vi "WaveformSimulator.vi"() -> ()   [LabVIEW 2015]
uses:
  <vilib>/imath/engines/lvmath2/RunTimeEngine/Managers/WorkSpace/UID Generator.vi
  <vilib>/imath/engines/lvmath2/RunTimeEngine/RunTimeType/NIMS_RunTimeType_From StrictType (excl LVString).vi
  <instcachedir>/0/NIMS_RunTimeType_From StrictType (excl LVString)_EB1C38A9BC5048DA9ABDA8F781E54D21.lvgen/NIMS_RunTimeType_From StrictType (excl LVString)_EB1C38A9BC5048DA9ABDA8F781E54D21_000.vi
  <vilib>/imath/engines/lvmath2/RunTimeEngine/LocalVariableDefStatement/MC_LocalVariableDefStatement_Display.vi
  <vilib>/imath/engines/lvmath2/RunTimeEngine/RangeToken/NIMS_Range.vi
  <instcachedir>/0/NIMS_Range_D919CC09935940E88F755EC1C6F49AC1.lvgen/NIMS_Range_D919CC09935940E88F755EC1C6F49AC1_000.vi
  <vilib>/imathl/engines/lvmath/Functions/Error Handling/Create Error.vi
  <vilib>/imath/engines/lvmath2/RunTimeEngine/ArithmeticOperatorToken/NIMS_ArithmeticOperator_plus.vi
  <instcachedir>/0/NIMS_ArithmeticOperator_plus_A4F2756F5ADB4A0090E0DBD7C10701C8.lvgen/NIMS_ArithmeticOperator_plus_A4F2756F5ADB4A0090E0DBD7C10701C8_004.vi
  <vilib>/imath/engines/lvmath2/RunTimeEngine/BuiltInFunctions/gensignal/NIMS_gensignal(str,RS,RS,RS).vi
  <vilib>/imath/engines/lvmath2/RunTimeEngine/BuiltInFunctions/linramp/NIMS_linramp.vi
  <vilib>/imath/engines/lvmath2/RunTimeEngine/VariableToken/NIMS_VariableToken_CondDefined.vi
  <instcachedir>/0/NIMS_VariableToken_CondDefined_FE30D0A1BFB24F098D41DEBABFE96BE1.lvgen/NIMS_VariableToken_CondDefined_FE30D0A1BFB24F098D41DEBABFE96BE1_001.vi
  <vilib>/imath/engines/lvmath2/RunTimeEngine/NodeEndStatement/NIMS_NodeEndStatement_Get Vector.vi
  <instcachedir>/0/NIMS_NodeEndStatement_Get Vector_ED7FC4F6B50246F79D573C75B2E51AF8.lvgen/NIMS_NodeEndStatement_Get Vector_ED7FC4F6B50246F79D573C75B2E51AF8_001.vi
  <vilib>/imath/engines/lvmath/Functions/Error Handling/MergeErrorsWrapper.vi
  <vilib>/imath/engines/lvmath2/RunTimeEngine/Managers/SymbolTable/Clear UID.vi
  <vilib>/imath/engines/lvmath2/RunTimeEngine/NodeEndStatement/NIMS_NodeEndStatement_Output.vi
  <instcachedir>/0/NIMS_NodeEndStatement_Output_53EC0D466D134D7ABD903AC30B43404B.lvgen/NIMS_NodeEndStatement_Output_53EC0D466D134D7ABD903AC30B43404B_005.vi
  <vilib>/imath/engines/lvmath2/RunTimeEngine/ErrorHandling/NIMS_Finalize Error.vi
  <vilib>/imath/engines/lvmath2/RunTimeEngine/Managers/SymbolTable/NIMS_WorkSpace.lvlib
panel:
  out "Waveform Output":cluster{"Time":dbl[], "Displacement":dbl[]} {"Displacement" format="%#_13g"; "Time" format="%#_13g"}
  in  "Waveform Parameters":T1
  in  "Digitizing Parameters":T2
  out "XY Graph":cluster{"t":dbl[], "x":dbl[]}(graph)
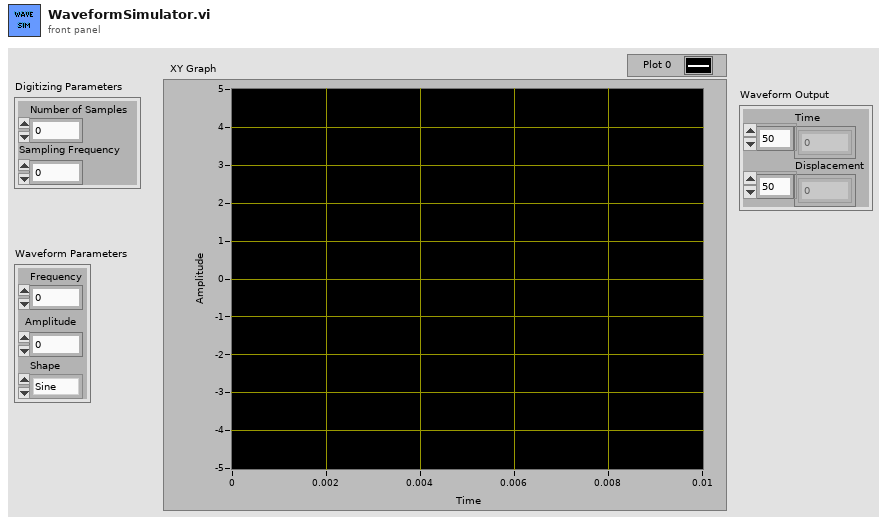
[diagram p1: front panel]
types:
  T1 = cluster{"Frequency":i32, "Amplitude":i32, "Shape":enum16{"Sine", "Cosine", "LinRamp", "Square", "SineCosine"}}
  T2 = cluster{"Number of Samples":i32, "Sampling Frequency":i32}
  T3 = enum16{"Sine", "Cosine", "LinRamp", "Square", "SineCosine"}
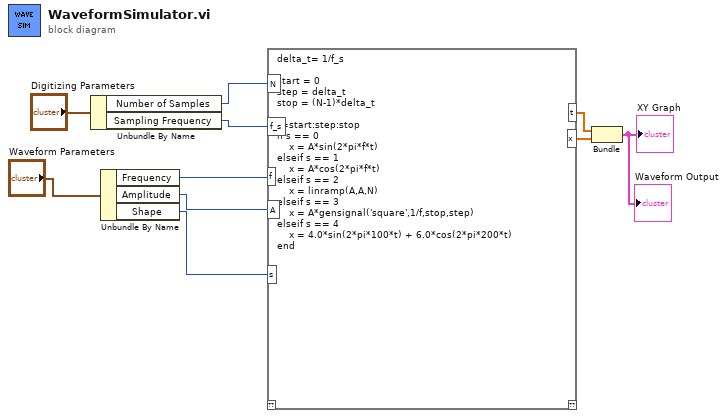
[diagram p0: block diagram]
diagram:
  n1 = Unbundle By Name("Digitizing Parameters") -> ("Number of Samples"=w7:i32, "Sampling Frequency"=w5:i32)
  n2 = Unbundle By Name("Waveform Parameters") -> ("Frequency"=w4:i32, "Amplitude"=w3:i32, "Shape"=w2:T3)
  n3 = mathscript code="delta_t= 1/f_s\n\nstart = 0\nstep = delta_t\nstop = (N-1)*delta_t\n\nt=start:step:stop\nif s == 0\n    x = A*sin(2*pi*f*t)\nelseif s == 1\n    x = A*cos(2*pi*f*t)\nelseif s == 2\n    x = linramp(A,A,N)\nelseif s == 3\n    x = A*gensignal('square',1/f,stop,step)\nelseif s == 4\n    x = 4.0*sin(2*pi*100*t) + 6.0*cos(2*pi*200*t)\nend"("N"=w7, "f"=w4, "A"=w3, "s"=w2, "f_s"=w5) -> ("t"=w10:dbl[], "x"=w9:dbl[])  [unwired: 1 in, 1 out]
  n4 = Bundle("t"=w10, "x"=w9) -> (→"XY Graph" →"Waveform Output":cluster{"t":dbl[], "x":dbl[]})  [unwired: 1 in]
